vi "Test.vi"   [LabVIEW 2019]
doc: "This VI is called when test mode begins, and will automatically be terminated when it ends. You can add manual or automatic tests and invoke them from the dashboard."
uses:
  Robot Global Data.vi
  <vilib>/Rock Robotics/Network Tables/NT Read Number.vi
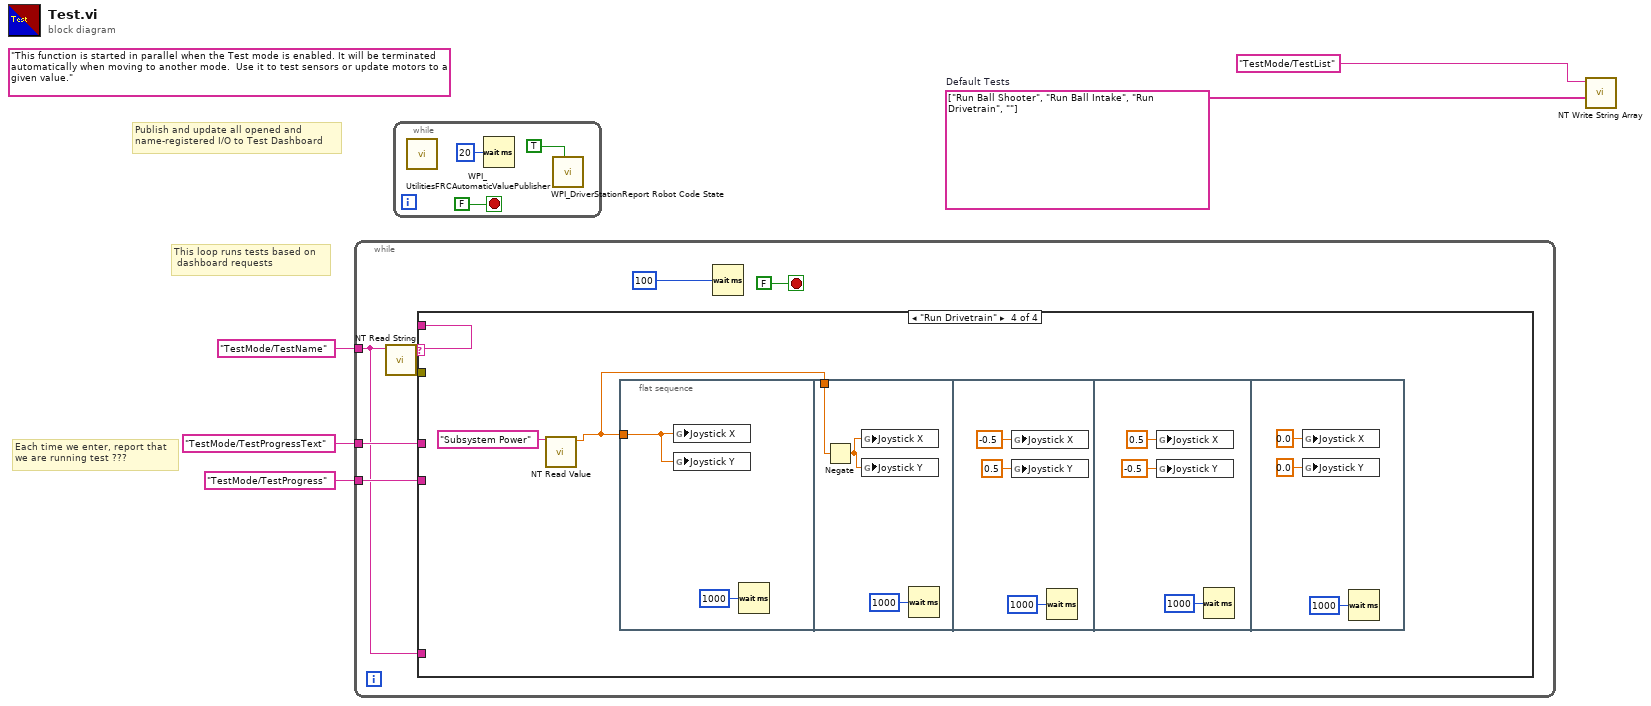
[diagram p0: block diagram]
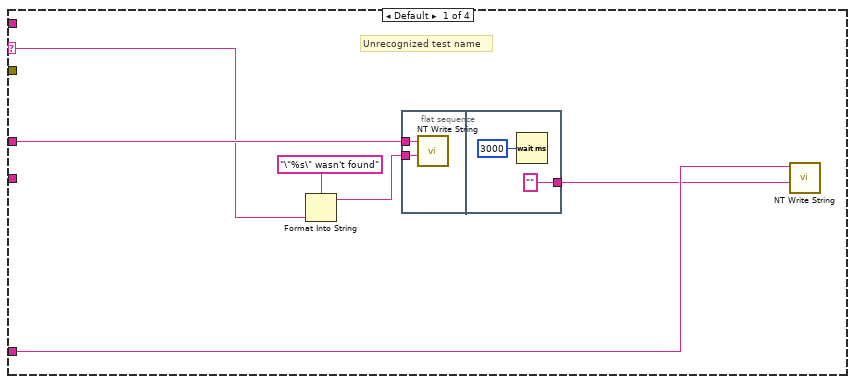
[diagram p2: hidden frame]
diagram:
  w2 = string[] ["Run Ball Shooter", "Run Ball Intake", "Run Drivetrain", ""]  # Default Tests
  (unwired) "This function is started in parallel when the Test mode is enabled. It will be terminated automatically when moving to another mode.  Use it to test sensors or update motors to a given value."
  # "This loop runs tests based on \n dashboard requests"
  # "Publish and update all opened and\nname-registered I/O to Test Dashboard"
  # "Each time we enter, report that\nwe are running test ???"
  n1 = while {
    tunnel: "TestMode/TestName" ("Name") -> [w7]
    tunnel: "TestMode/TestProgressText" ("Name") -> [w10]
    tunnel: "TestMode/TestProgress" ("Name") -> [w9]
    stop <- FALSE stop-if-true
    n2 = call <vilib>:"NT Read String.vi"("Name"=w7) -> ("error out"=w6:errorcluster, "String"=w8:string)  [unwired: 9 in]
    n3 = case shown="\"Run Drivetrain\"" w8 {
      selector: w8 -> [w17 _ _ _]
      tunnel: w7 -> [w14 _ _ _]
      tunnel: w10 -> [w18 _ _ _]
      tunnel: w9 -> [_ _ _ _]
      tunnel: w8 -> [_ _ _ _]
      tunnel: w6 -> [_ _ _ _]
      frame Default {
        # "Unrecognized test name"
        n4 = Format Into String(format string="\"%s\" wasn't found" ("Name"), w17) -> (resulting string=w16:string)  [unwired: 2 in, 1 out]
        n5 = flat-sequence {
          tunnel: w18 -> [w19]
          tunnel: w16 -> [w20]
          tunnel: ["" ("Name")] -> w13
          frame #0 {
            n6 = call <vilib>:"NT Write String.vi"("String"=w20, "Name"=w19) -> ()  [unwired: 9 in, 1 out]
          }
          frame #1 {
            n7 = Wait (ms)(milliseconds to wait=u32 3000) -> ()  [unwired: 1 out]
          }
        }
        n8 = call <vilib>:"NT Write String.vi"("String"=w13, "Name"=w14) -> ()  [unwired: 9 in, 1 out]
      }
      frame "Run Ball Shooter" {
      }
      frame "Run Ball Intake" {
      }
      frame "Run Drivetrain" {
        n9 = call-poly <vilib>:"NT Read Value.vi"("Name"="Subsystem Power") -> ("Numeric"=w23:dbl)  [unwired: 9 in, 1 out]
        n10 = flat-sequence {
          tunnel: w23 -> [w25]
          tunnel: w23 -> [w27]
          frame #0 {
            n11 = global write "Robot Global Data.vi" "Joystick X"(w25) -> ()
            n12 = global write "Robot Global Data.vi" "Joystick Y"(w25) -> ()
            n13 = Wait (ms)(milliseconds to wait=u32 1000) -> ()  [unwired: 1 out]
          }
          frame #1 {
            n14 = Negate(x=w27) -> (-x=w28:dbl)
            n15 = global write "Robot Global Data.vi" "Joystick X"(w28) -> ()
            n16 = global write "Robot Global Data.vi" "Joystick Y"(w28) -> ()
            n17 = Wait (ms)(milliseconds to wait=u32 1000) -> ()  [unwired: 1 out]
          }
          frame #2 {
            n18 = global write "Robot Global Data.vi" "Joystick X"(-0.5 ("Joystick X")) -> ()
            n19 = global write "Robot Global Data.vi" "Joystick Y"(0.5 ("Joystick Y")) -> ()
            n20 = Wait (ms)(milliseconds to wait=u32 1000) -> ()  [unwired: 1 out]
          }
          frame #3 {
            n21 = global write "Robot Global Data.vi" "Joystick X"(0.5 ("Joystick X")) -> ()
            n22 = global write "Robot Global Data.vi" "Joystick Y"(-0.5 ("Joystick Y")) -> ()
            n23 = Wait (ms)(milliseconds to wait=u32 1000) -> ()  [unwired: 1 out]
          }
          frame #4 {
            n24 = global write "Robot Global Data.vi" "Joystick X"(0.0 ("Joystick X")) -> ()
            n25 = global write "Robot Global Data.vi" "Joystick Y"(0.0 ("Joystick Y")) -> ()
            n26 = Wait (ms)(milliseconds to wait=u32 1000) -> ()  [unwired: 1 out]
          }
        }
      }
    }
    n27 = Wait (ms)(milliseconds to wait=u32 100) -> ()  [unwired: 1 out]
  }
  n28 = while {
    stop <- FALSE stop-if-true
    n29 = call <vilib>:"WPI_UtilitiesFRCAutomaticValuePublisher.vi"() -> ()  [unwired: 12 in]
    n30 = Wait (ms)(milliseconds to wait=u32 20) -> ()  [unwired: 1 out]
    n31 = call <vilib>:"WPI_DriverStationReport Robot Code State.vi"("Test"=TRUE ("Autonomous")) -> ()  [unwired: 10 in, 1 out]
  }
  n32 = call <vilib>:"NT Write String Array.vi"("String Array"=w2, "Name"="TestMode/TestList") -> ()  [unwired: 9 in, 1 out]
